vi "CAA.vi"(10 "Process Variable":dbl, 11 "Setpoint":dbl) -> (2 "Output":dbl)   [LabVIEW 2014]
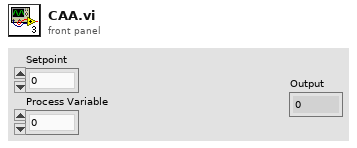
[diagram p1: front panel]
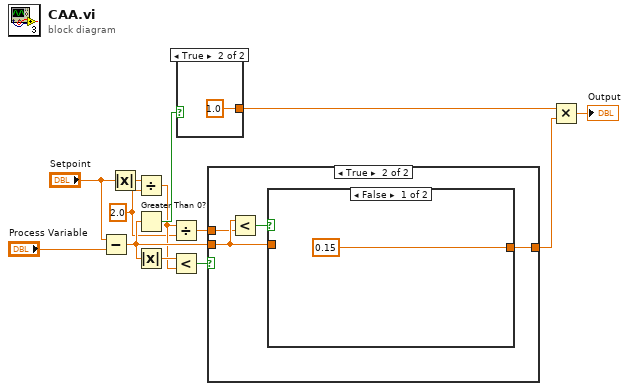
[diagram p0: block diagram]
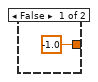
[diagram p2: hidden frame]
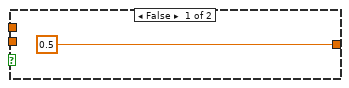
[diagram p3: hidden frame]
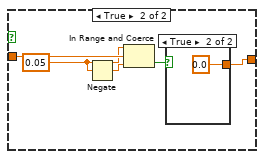
[diagram p4: hidden frame]
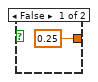
[diagram p5: hidden frame]
diagram:
  w4 = 2.0 ("y")
  n1 = Subtract(x="Setpoint", y="Process Variable") -> (x-y=w10:dbl)
  n2 = Absolute Value(x="Setpoint") -> (abs(x)=w2:dbl)
  n3 = Divide(x=w2, y=w4) -> (x/y=w5:dbl)
  n4 = Greater Than 0?(x=w10) -> (x > 0?=w9:bool)
  n5 = Absolute Value(x=w10) -> (abs(x)=w11:dbl)
  n6 = Divide(x=w5, y=w4) -> (x/y=w3:dbl)
  n7 = Less?(x=w11, y=w5) -> (x < y?=w12:bool)
  n8 = case shown="True" w9 {
    tunnel: [-1.0 1.0] -> w6
    frame False {
    }
    frame True {
    }
  }
  n9 = case shown="True" w12 {
    tunnel: w10 -> [_ w19]
    tunnel: [0.5 w18] -> w7
    tunnel: w3 -> [_ w17]
    frame False {
    }
    frame True {
      n10 = Less?(x=w19, y=w17) -> (x < y?=w20:bool)
      n11 = case shown="False" w20 {
        tunnel: w19 -> [_ w25]
        tunnel: [0.15 w22] -> w18
        frame False {
        }
        frame True {
          w23 = 0.05 ("Tolerance")
          n12 = Negate(x=w23) -> (-x=w24:dbl)
          n13 = In Range and Coerce(upper limit=w23, x=w25, lower limit=w24) -> (In Range?=w26:bool)  [unwired: 1 out]
          n14 = case shown="True" w26 {
            tunnel: [0.25 0.0] -> w22
            frame False {
            }
            frame True {
            }
          }
        }
      }
    }
  }
  n15 = Multiply(x=w6, y=w7) -> (x*y=→"Output":dbl)
